vi "多从板对应参数-new.vi"(2 "从板个数":dbl=1.0) -> (0 "输出数组":string[](array[string]))   [LabVIEW 2013]
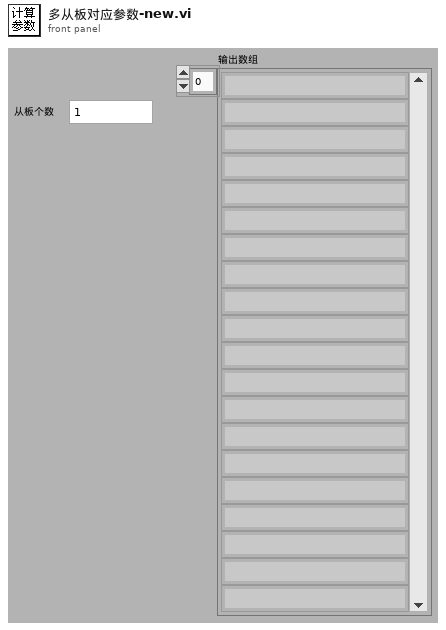
[diagram p1: front panel]
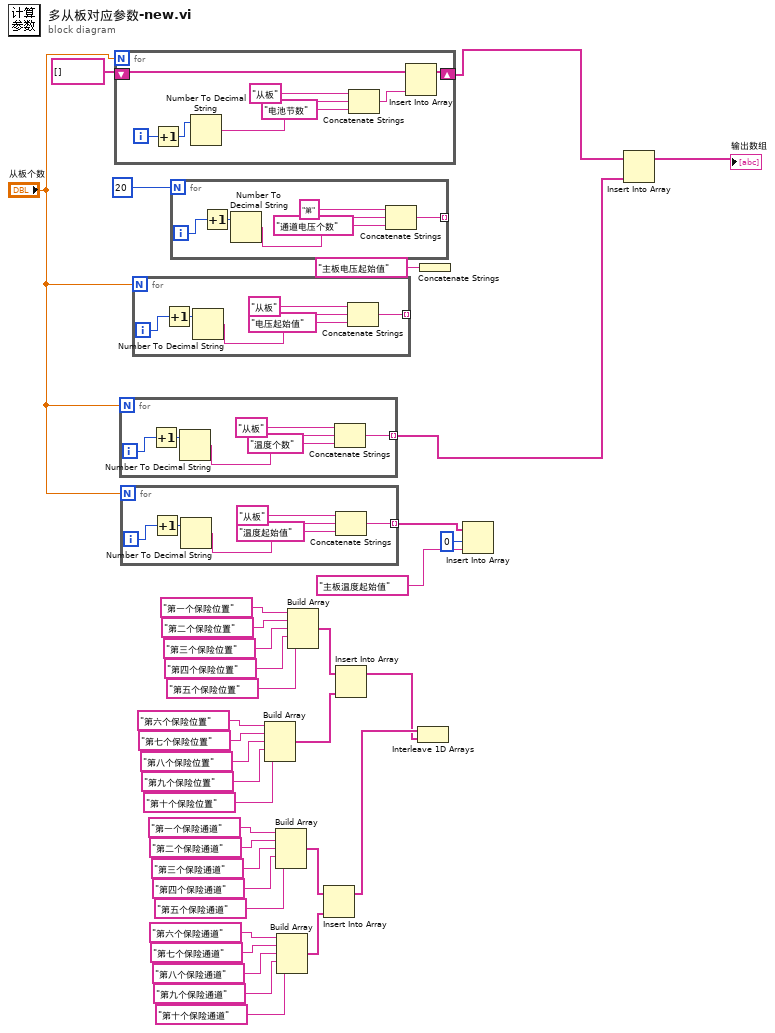
[diagram p0: block diagram]
diagram:
  n1 = for {
    N: "从板个数" -> [_]
    shift-right: [w41] -> w2
    shift-left: string[] [] -> [w40]
    i -> [w39]
    n2 = Increment(x=w39) -> (x+1=w37:i32)
    n3 = Number To Decimal String(number=w37) -> (decimal integer string=w43:string)  [unwired: 1 out]
    n4 = Concatenate Strings("从板" ("字符串"), w43, "电池节数" ("字符串")) -> (w38:string)
    n5 = Insert Into Array(array=w40, new element=w38) -> (w41:string[])  [unwired: 1 in]
  }
  n6 = for {
    N: "从板个数" -> [_]
    tunnel: [w45] -> w1 mode=indexing
    i -> [w50]
    n7 = Increment(x=w50) -> (x+1=w49:i32)
    n8 = Number To Decimal String(number=w49) -> (decimal integer string=w47:string)  [unwired: 1 out]
    n9 = Concatenate Strings("从板" ("字符串"), w47, "温度个数" ("字符串")) -> (w45:string)
  }
  n10 = for {
    N: "从板个数" -> [_]
    tunnel: [w51] -> w30 mode=indexing
    i -> [w56]
    n11 = Increment(x=w56) -> (x+1=w55:i32)
    n12 = Number To Decimal String(number=w55) -> (decimal integer string=w53:string)  [unwired: 1 out]
    n13 = Concatenate Strings("从板" ("字符串"), w53, "温度起始值" ("字符串")) -> (w51:string)
  }
  n14 = for {
    N: "从板个数" -> [_]
    tunnel: [w57] -> _ mode=indexing
    i -> [w62]
    n15 = Increment(x=w62) -> (x+1=w61:i32)
    n16 = Number To Decimal String(number=w61) -> (decimal integer string=w59:string)  [unwired: 1 out]
    n17 = Concatenate Strings("从板" ("字符串"), w59, "电压起始值" ("字符串")) -> (w57:string)
  }
  n18 = for {
    N: 20 -> [_]
    tunnel: [w63] -> _ mode=indexing
    i -> [w68]
    n19 = Increment(x=w68) -> (x+1=w67:i32)
    n20 = Number To Decimal String(number=w67) -> (decimal integer string=w65:string)  [unwired: 1 out]
    n21 = Concatenate Strings("第" ("字符串"), w65, "通道电压个数" ("字符串")) -> (w63:string)
  }
  n22 = Build Array("第六个保险位置" ("字符串"), "第七个保险位置" ("字符串"), "第八个保险位置" ("字符串"), "第九个保险位置" ("字符串"), "第十个保险位置" ("字符串")) -> (w17:string[])
  n23 = Build Array("第一个保险通道" ("字符串"), "第二个保险通道" ("字符串"), "第三个保险通道" ("字符串"), "第四个保险通道" ("字符串"), "第五个保险通道" ("字符串")) -> (w6:string[])
  n24 = Build Array("第六个保险通道" ("字符串"), "第七个保险通道" ("字符串"), "第八个保险通道" ("字符串"), "第九个保险通道" ("字符串"), "第十个保险通道" ("字符串")) -> (w5:string[])
  n25 = Build Array("第一个保险位置" ("字符串"), "第二个保险位置" ("字符串"), "第三个保险位置" ("字符串"), "第四个保险位置" ("字符串"), "第五个保险位置" ("字符串")) -> (w18:string[])
  n26 = Insert Into Array(array=w6, new element=w5) -> (w4:string[])  [unwired: 1 in]
  n27 = Insert Into Array(array=w18, new element=w17) -> (w3:string[])  [unwired: 1 in]
  n28 = Interleave 1D Arrays(w4, w3) -> ()  [unwired: 1 out]
  n29 = Concatenate Strings("主板电压起始值" ("字符串")) -> ()  [unwired: 1 out]
  n30 = Insert Into Array(array=w30, index=0 ("索引"), new element="主板温度起始值" ("字符串")) -> ()  [unwired: 1 out]
  n31 = Insert Into Array(array=w2, new element=w1) -> (→"输出数组":string[])  [unwired: 1 in]
